vi "TCP Writer.vi"(1 "occurrence":refnum<k4>) -> (0 "stopped":bool)   [LabVIEW 2013]
uses:
  Device Driver/shared/stop FGV control.ctl
panel:
  in  "error in":errorcluster
  out "time for sending TCP":u32(graph)
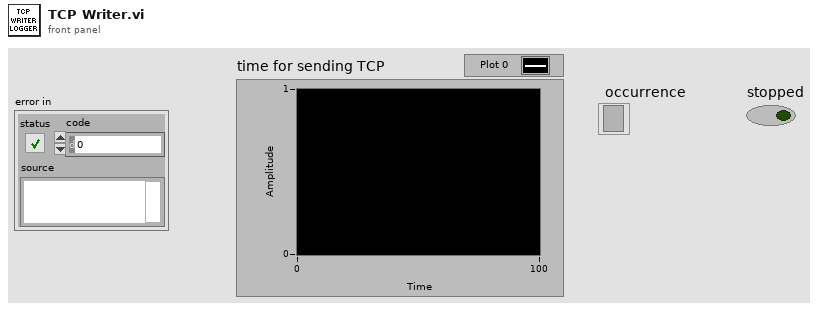
[diagram p1: front panel]
types:
  T1 = typedef "stop FGV control.ctl" = enum16{"Clear", "Write", "Read"}
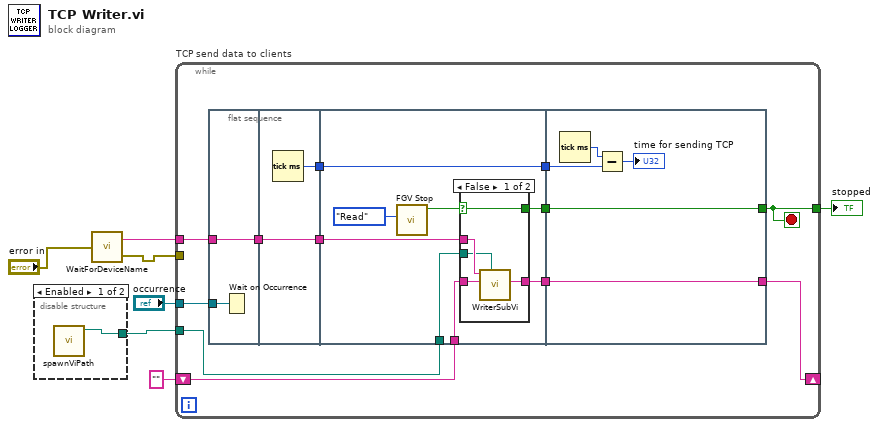
[diagram p0: block diagram]
diagram:
  n1 = disable-structure shown="Enabled" {
    disable-tunnel: [w8 _] -> w7
    frame Enabled {
      n2 = call "spawnViPath.vi"() -> ("Spawn vi path"=w8:path)  [unwired: 10 in, 1 out]
    }
    frame Disabled {
    }
  }
  n3 = call "WaitForDeviceName.vi"("error in 2"="error in") -> ("Device Name"=w5:string, "error in"=w4:errorcluster)
  n4 = while "TCP send data to clients" {
    tunnel: "occurrence" -> [w20]
    tunnel: [w19] -> w2
    tunnel: w4 -> [_]
    tunnel: w5 -> [w18]
    shift-right: [w17] -> _
    shift-left: "" ("head buffer out") -> [w16]
    tunnel: w7 -> [w9]
    stop <- w19 stop-if-true
    n5 = flat-sequence {
      tunnel: w20 -> [w22]
      tunnel: w18 -> [w21]
      tunnel: [w21] -> w15
      tunnel: w15 -> [w24]
      tunnel: [w24] -> w14
      tunnel: [w23] -> w11
      tunnel: w14 -> [w30]
      tunnel: w16 -> [w28]
      tunnel: [w31] -> w13
      tunnel: [w29] -> w12
      tunnel: w11 -> [w27]
      tunnel: [w27] -> w10
      tunnel: w9 -> [w26]
      tunnel: [w43] -> w17
      tunnel: [w44] -> w19
      tunnel: w13 -> [w44]
      tunnel: w12 -> [w43]
      tunnel: w10 -> [w41]
      frame #0 {
        n6 = Wait on Occurrence(2:w22) -> ()  [unwired: 2 in, 1 out]
      }
      frame #1 {
        n7 = Tick Count (ms)() -> (millisecond timer value=w23:u32)
      }
      frame #2 {
        n8 = call "FGV Stop.vi"("Function"=stop_FGV_control."Read") -> ("stop out"=w32:bool)  [unwired: 9 in, 1 out]
        n9 = case shown="False" w32 {
          selector: w32 -> [w37 w39]
          tunnel: [w37 w39] -> w31
          tunnel: w30 -> [w36 _]
          tunnel: [w35 w38] -> w29
          tunnel: w28 -> [w34 w38]
          tunnel: w26 -> [w33 _]
          frame False {
            n10 = call "WriterSubVi.vi"("Spawn vi path"=w33, "head buffer"=w34, "Device Name"=w36) -> ("head buffer out"=w35:string)  [unwired: 7 in, 1 out]
          }
          frame True {
          }
        }
      }
      frame #3 {
        n11 = Tick Count (ms)() -> (millisecond timer value=w42:u32)
        n12 = Subtract(x=w42, y=w41) -> (x-y=→"time for sending TCP":u32)
      }
    }
  }
  "stopped" <- w2
